vi "GenerateMove.vi"(3 "Error in":errorcluster, 4 "Formatted input string":string, 5 "Input Array":dbl[](array[numeric])) -> (0 "Error out":errorcluster, 1 "Output Array":dbl[](array[numeric]), 2 "Formatted output string":string)   [LabVIEW 2011]
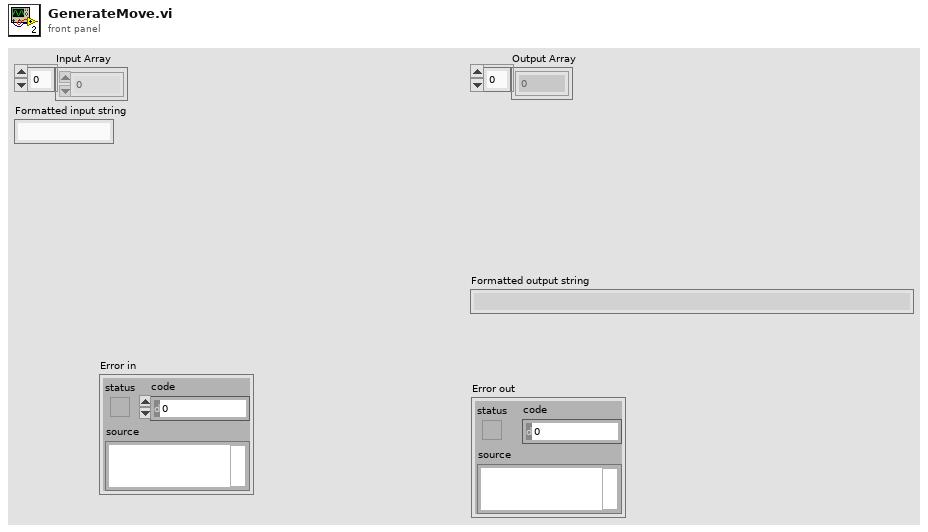
[diagram p1: front panel]
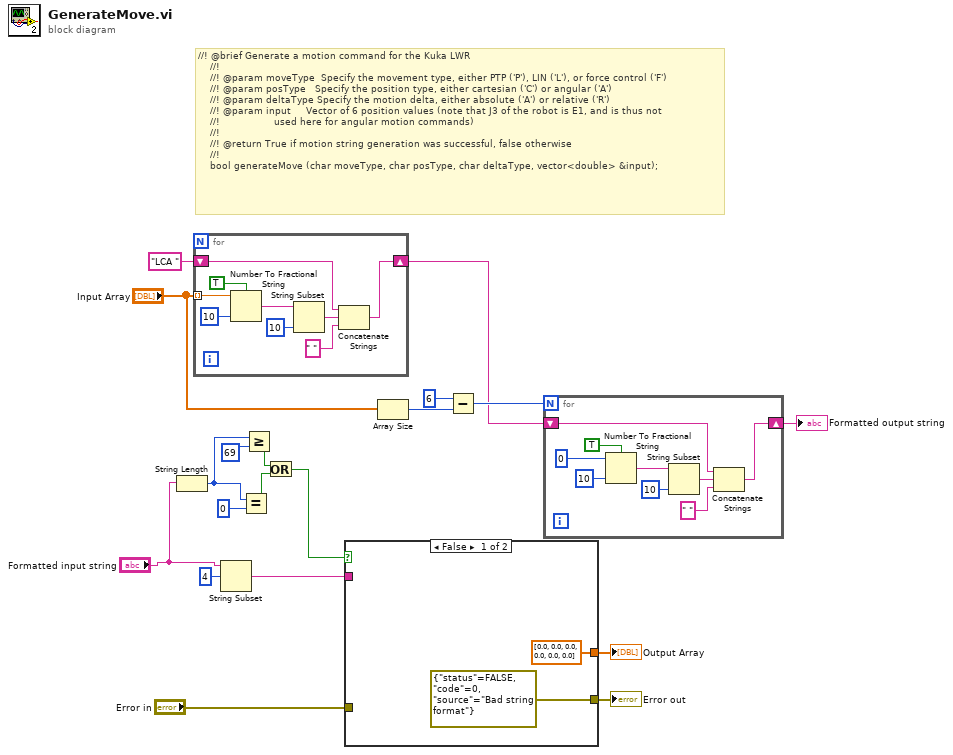
[diagram p0: block diagram]
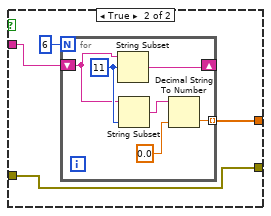
[diagram p2: hidden frame]
diagram:
  # "//! @brief Generate a motion command for the Kuka LWR\n    //!\n    //! @param moveType  Specify the movement type, either PTP ('P'), LIN ('L'), or force control ('F')\n    //! @param posType   Specify the position type, either cartesian ('C') or angular ('A')\n    //! @param deltaType Specify the motion delta, either absolute ('A') or relative ('R')\n    //! @param input     Vector of 6 position values (note that J3 of the robot is E1, and is thus not\n    //!                  used here for angular motion commands)\n    //!\n    //! @return True if motion string generation was successful, false otherwise\n    //!\n    bool generateMove (char moveType, char posType, char deltaType, vector<double> &input);"
  n1 = String Length(string="Formatted input string") -> (length=w9:i32)
  n2 = for {
    tunnel: "Input Array" -> [w28] mode=indexing
    shift-right: [w20] -> w15
    shift-left: "LCA " ("F-format string") -> [w23]
    n3 = Number To Fractional String(use system decimal point (T)=TRUE, number=w28, precision (6)=i16 10) -> (F-format string=w24:string)  [unwired: 1 in]
    n4 = String Subset(string=w24, length (rest)=10 ("length (rest)")) -> (substring=w22:string)  [unwired: 1 in]
    n5 = Concatenate Strings(w23, w22, " " ("F-format string")) -> (w20:string)
  }
  n6 = String Subset(string="Formatted input string", offset (0)=4) -> (substring=w4:string)  [unwired: 1 in]
  n7 = Equal?(x=w9, y=0) -> (x = y?=w6:bool)
  n8 = Greater Or Equal?(x=w9, y=69) -> (x >= y?=w7:bool)
  n9 = Or(x=w7, y=w6) -> (x .or. y?=w5:bool)
  n10 = case shown="False" w5 {
    tunnel: w4 -> [_ w33]
    tunnel: [dbl[] [0.0, 0.0, 0.0, 0.0, 0.0, 0.0] w32] -> w2
    tunnel: [errorcluster {"status"=FALSE, "code"=0, "source"="Bad string format"} ("error constant") w31] -> w1
    tunnel: "Error in" -> [_ w31]
    frame False {
    }
    frame True {
      n11 = for {
        N: 6 -> [_]
        shift-right: [w40] -> _
        shift-left: w33 -> [w38]
        tunnel: [w35] -> w32 mode=indexing
        w39 = 11 ("offset (0)")
        n12 = String Subset(string=w38, offset (0)=w39) -> (substring=w40:string)  [unwired: 1 in]
        n13 = String Subset(string=w38, length (rest)=w39) -> (substring=w37:string)  [unwired: 1 in]
        n14 = Decimal String To Number(string=w37, default (0L)=0.0 ("default (0 I32)")) -> (number=w35:dbl)  [unwired: 1 in, 1 out]
      }
    }
  }
  "Output Array" <- w2
  "Error out" <- w1
  n15 = Array Size(array="Input Array") -> (size(s)=w17:i32)
  n16 = Subtract(x=i16 6 ("precision (6)"), y=w17) -> (x-y=w16:i32)
  n17 = for {
    N: w16 -> [_]
    shift-right: [w42] -> w12
    shift-left: w15 -> [w45]
    n18 = Number To Fractional String(use system decimal point (T)=TRUE, number=i16 0 ("precision (6)"), precision (6)=i16 10) -> (F-format string=w46:string)  [unwired: 1 in]
    n19 = String Subset(string=w46, length (rest)=10 ("length (rest)")) -> (substring=w44:string)  [unwired: 1 in]
    n20 = Concatenate Strings(w45, w44, " " ("F-format string")) -> (w42:string)
  }
  "Formatted output string" <- w12
